vi "Create G Plugin.vi"() -> ()   [LabVIEW 2021, in "G Plugin Editor.lvlib"]
uses:
  _Editor/G Plugin Editor.lvlib
  <vilib>/Utility/error.llb/ErrWarn.ctl
  _Editor/controls/Data Holder.ctl
  _Editor/NI_AB_API_PPL_Extensions/NI_AB_API_PPL_Extensions.lvclass
panel:
  in  "Group":string caption="G Plug-in Group"
  in  "Plugin Type":string
  out "Status":T1=TRUE caption="Plug-in name must be unique and cannot contain any of the following characters:\n           \\ / : * ? \" < > |"
  in  "Create Measurement Service":bool
  in  "Name":string caption="G Plug-in Name"
  out "Active Project Name":string
  # "* Project in which the InstrumentStudio G plug-in will be created"
  # "* Category under which the plug-in will be populated under\n   InstrumentStudio Edit Layout Dialog"
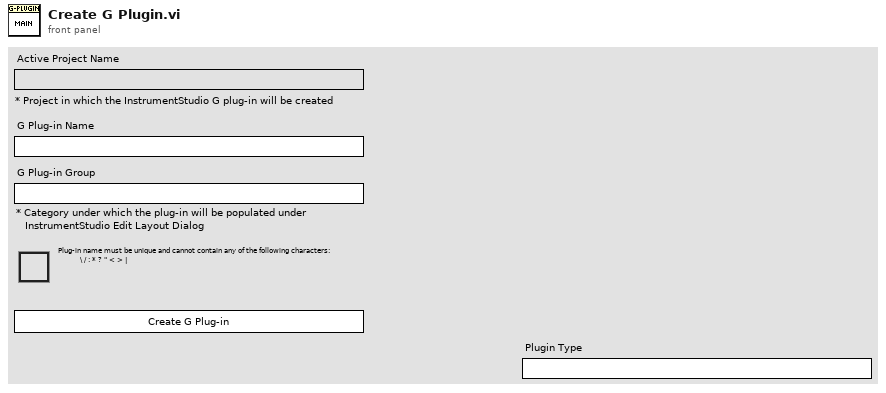
[diagram p1: front panel]
types:
  T1 = typedef "ErrWarn.ctl" = bool
  T2 = typedef "G Plugin Editor.lvlib/Data Holder.ctl" = cluster{"project ref":refnum<vi>, "Name":string, "Plugin Type":string, "Plugin Group Name":string}
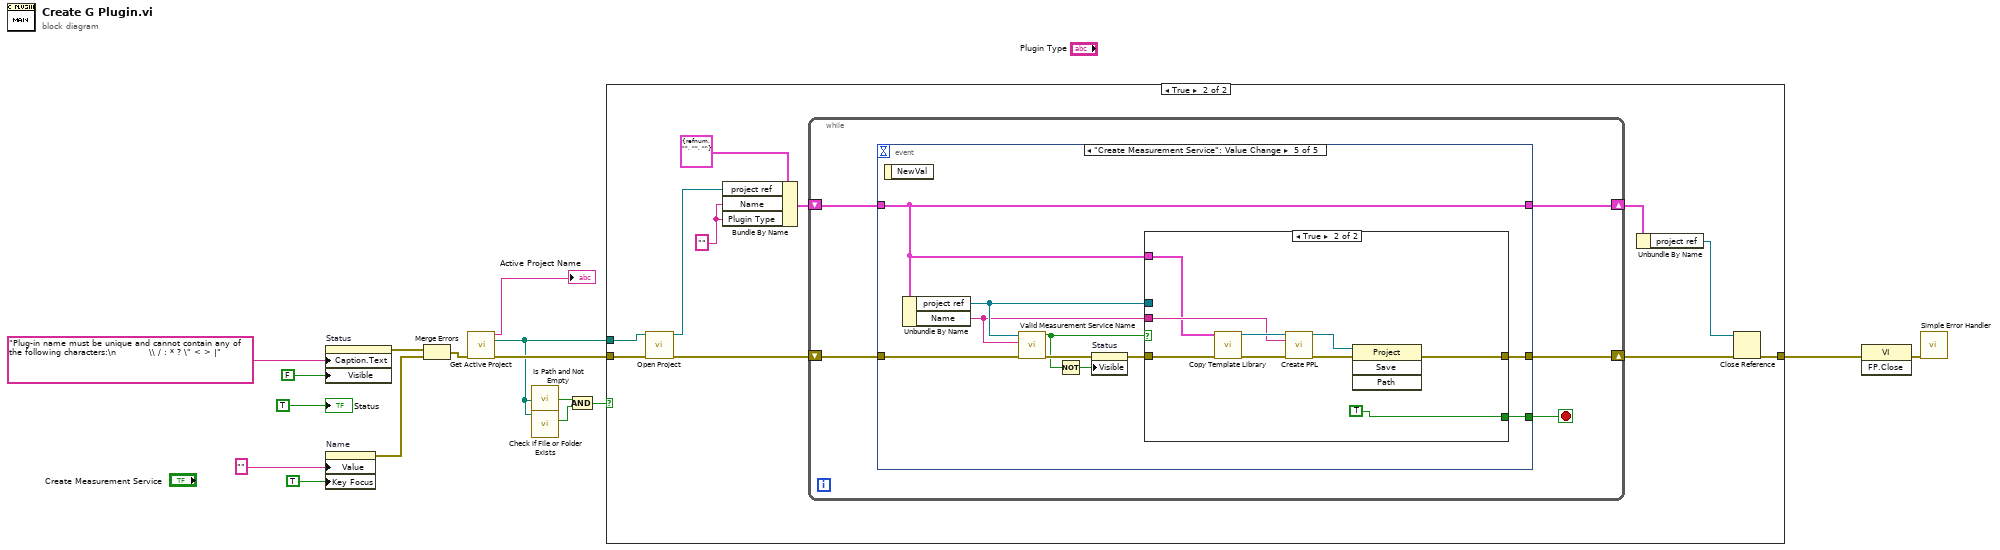
[diagram p0: block diagram]
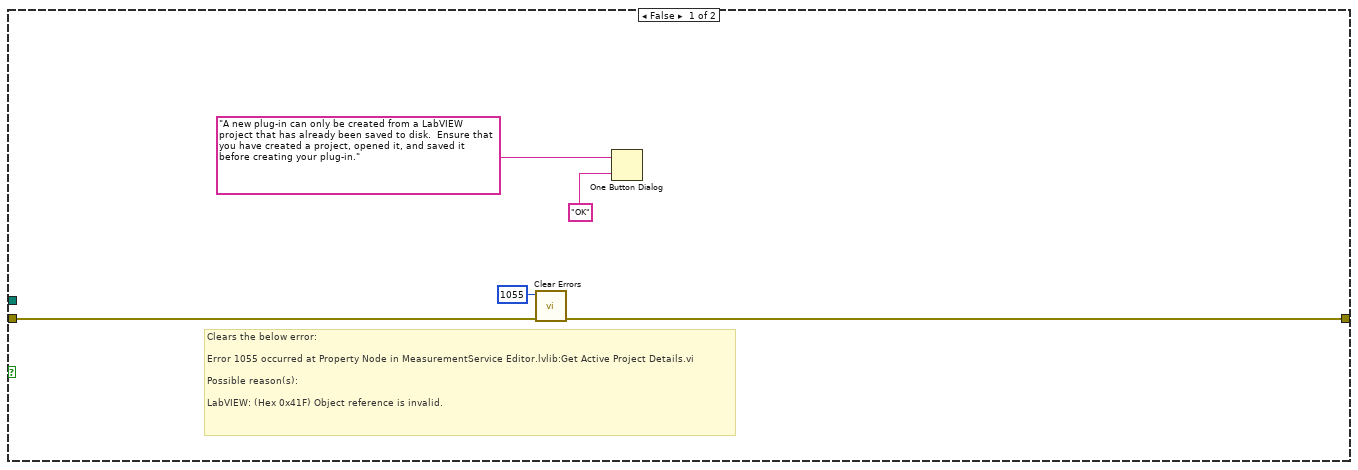
[diagram p2: hidden frame]
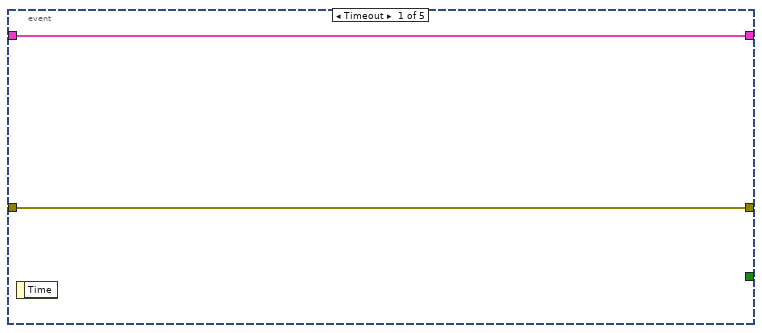
[diagram p3: hidden frame]
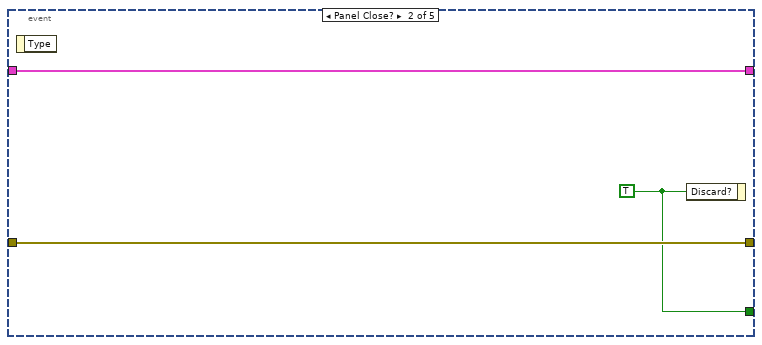
[diagram p4: hidden frame]
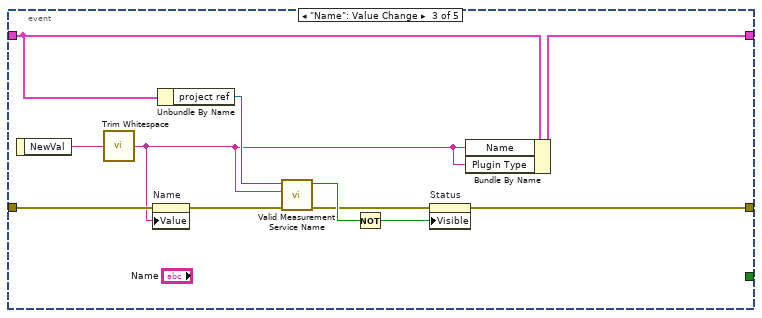
[diagram p5: hidden frame]
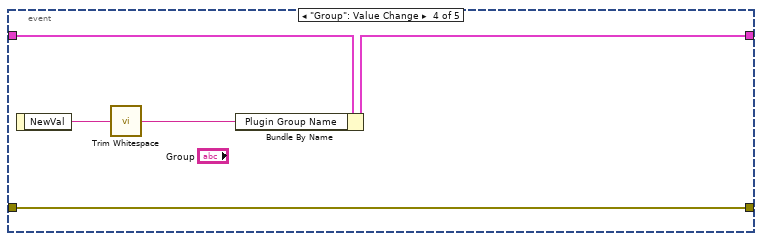
[diagram p6: hidden frame]
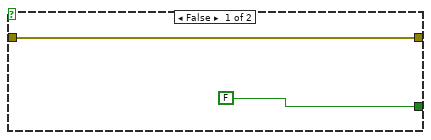
[diagram p7: hidden frame]
diagram:
  n1 = property on="Status" class="Bool"("Caption.Text"="Plug-in name must be unique and cannot contain any of the following characters:\n           \\ / : * ? \" < > |" ("Status"), "Visible"=FALSE) -> (error out=w11:errorcluster)  [unwired: 2 in, 1 out]
  n2 = property on="Name" class="Str"("Value"="" ("InstrumentStudio G Plug-in Name"), "Key Focus"=TRUE) -> (error out=w10:errorcluster)  [unwired: 2 in, 1 out]
  n3 = Merge Errors(w11, w10) -> (w9:errorcluster)
  n4 = call "Get Active Project.vi"("error in"=w9) -> ("name"=→"Active Project Name":string, "path"=w2:path, "error out"=w6:errorcluster)  [unwired: 12 in]
  n5 = call <vilib>:"Is Path and Not Empty.vi"("path"=w2) -> ("Is Path and Not Empty?"=w7:bool)  [unwired: 4 in]
  n6 = call <vilib>:"Check if File or Folder Exists.vi"("path"=w2) -> ("file or folder exists?"=w8:bool)  [unwired: 8 in, 2 out]
  n7 = And(x=w7, y=w8) -> (x .and. y?=w5:bool)
  n8 = case shown="True" w5 {
    tunnel: w6 -> [w18 w30]
    tunnel: [w17 w22] -> w3
    tunnel: w2 -> [_ w32]
    frame False {
      # "Clears the below error:\n\nError 1055 occurred at Property Node in MeasurementService Editor.lvlib:Get Active Project Details.vi\n\nPossible reason(s):\n\nLabVIEW: (Hex 0x41F) Object reference is invalid."
      n9 = call <vilib>:"Clear Errors.vi"("error in (no error)"=w18, "specific error code to clear (0: all)"=1055) -> ("error out"=w17:errorcluster)  [unwired: 4 in, 1 out]
      n10 = One Button Dialog(message="A new plug-in can only be created from a LabVIEW project that has already been saved to disk.  Ensure that you have created a project, opened it, and saved it before creating your plug-in.", button name ("OK")="OK") -> ()  [unwired: 1 out]
    }
    frame True {
      w26 = "" ("Name")
      n11 = call "Open Project.vi"("path"=w32, "error in"=w30) -> ("project ref"=w28:refnum<vi>, "error out"=w31:errorcluster)  [unwired: 12 in]
      n12 = Bundle By Name(cluster=T2 {"project ref"=refnum, "Name"="", "Plugin Type"="", "Plugin Group Name"=""}, "project ref"=w28, "Name"=w26, "Plugin Type"=w26) -> (w27:T2)
      n13 = while {
        shift-right: [w34] -> w23
        shift-left: w31 -> [w37]
        shift-right: [w35] -> w25
        shift-left: w27 -> [w36]
        stop <- w33 stop-if-true
        n14 = event shown="[4] \"Create Measurement Service\": Value Change" {
          selector: _ -> [_ _ _ _ _]
          dyn-events: _ -> [_ _ _ _ _]
          timeout: _ -> [_ _ _ _ _]
          tunnel: w37 -> [w38 w41 w44 w57 w68]
          tunnel: w36 -> [w39 w42 w51 w58 w59]
          tunnel: [w39 w42 w52 w55 w59] -> w35
          tunnel: [w38 w41 w48 w57 w63] -> w34
          tunnel: [_ w40 _ _ w60] -> w33
          event Timeout {
            n15 = event-data() -> ()  [unwired: 1 in, 1 out]
          }
          event Panel Close? {
            w40 = TRUE ("Discard?")
            n16 = event-data() -> ()  [unwired: 1 in, 1 out]
            n17 = event-data("Discard?"=w40) -> ()  [unwired: 1 in, 1 out]
          }
          event "Name": Value Change {
            n18 = event-data() -> ("NewVal"=w53:string)  [unwired: 1 in]
            n19 = call <vilib>:"Trim Whitespace.vi"("string"=w53) -> ("trimmed string"=w43:string)  [unwired: 1 in]
            n20 = property on="Name" class="Str"(error in=w44, "Value"=w43) -> (error out=w45:errorcluster)  [unwired: 1 in, 1 out]
            n21 = Unbundle By Name(w51) -> ("project ref"=w50:refnum<vi>)
            n22 = call "Valid Measurement Service Name.vi"("error in"=w45, "requested plugin name"=w43, "project ref"=w50) -> ("error out"=w47:errorcluster, "valid name?"=w49:bool)  [unwired: 7 in]
            n23 = Not(x=w49) -> (.not. x?=w46:bool)
            n24 = property on="Status" class="Bool"(error in=w47, "Visible"=w46) -> (error out=w48:errorcluster)  [unwired: 1 in, 1 out]
            n25 = Bundle By Name(cluster=w51, "Name"=w43, "Plugin Type"=w43) -> (w52:T2)
          }
          event "Group": Value Change {
            n26 = event-data() -> ("NewVal"=w56:string)  [unwired: 1 in]
            n27 = call <vilib>:"Trim Whitespace.vi"("string"=w56) -> ("trimmed string"=w54:string)  [unwired: 1 in]
            n28 = Bundle By Name(cluster=w58, "Plugin Group Name"=w54) -> (w55:T2)
          }
          event "Create Measurement Service": Value Change {
            n29 = event-data() -> ()  [unwired: 1 in, 1 out]
            n30 = Unbundle By Name(w59) -> ("project ref"=w62:refnum<vi>, "Name"=w61:string)
            n31 = call "Valid Measurement Service Name.vi"("error in"=w68, "requested plugin name"=w61, "project ref"=w62) -> ("error out"=w66:errorcluster, "valid name?"=w65:bool)  [unwired: 7 in]
            n32 = Not(x=w65) -> (.not. x?=w67:bool)
            n33 = property on="Status" class="Bool"(error in=w66, "Visible"=w67) -> (error out=w64:errorcluster)  [unwired: 1 in, 1 out]
            n34 = case shown="True" w65 {
              tunnel: w64 -> [w70 w79]
              tunnel: [w70 w72] -> w63
              tunnel: w62 -> [_ _]
              tunnel: w61 -> [_ w75]
              tunnel: [FALSE ("Discard?") TRUE ("Discard?")] -> w60
              tunnel: w59 -> [_ w71]
              frame False {
              }
              frame True {
                n35 = call "Copy Template Library.vi"("Configuration"=w71, "error in (no error)"=w79) -> ("project ref out"=w78:refnum<vi>, "error out"=w77:errorcluster)  [unwired: 12 in]
                n36 = call "Create PPL.vi"("Project Refnum"=w78, "Build specification name"=w75, "error in (no error)"=w77) -> ("project ref out"=w74:refnum<vi>, "error out"=w73:errorcluster)  [unwired: 10 in, 1 out]
                n37 = invoke class="Project" method="Save"(reference=w74, error in=w73) -> (error out=w72:errorcluster)  [unwired: 2 in, 3 out]
              }
            }
          }
        }
      }
      n38 = Unbundle By Name(w25) -> ("project ref"=w24:refnum<vi>)
      n39 = Close Reference(reference=w24, error in (no error)=w23) -> (error out=w22:errorcluster)
    }
  }
  n40 = invoke class="VI" method="FP.Close"(error in=w3) -> (error out=w4:errorcluster)  [unwired: 2 in, 2 out]
  n41 = call <vilib>:"Simple Error Handler.vi"("error in (no error)"=w4) -> ()  [unwired: 4 in, 5 out]
  "Status" <- T1 TRUE ("Status")
